vi "MDPtrMgr Info.vi"(8 "error in (no error)":errorcluster) -> (0 "error out":errorcluster, 1 "# free elements in queue":i32, 2 "# elements in queue":i32, 3 "Queue Names":string[](array[string]), 4 "#queues":i32)   [LabVIEW 2017, in "MDPtr.lvlib"]
uses:
  MDPtr.lvlib
  _MDPtrMgr/MDPtrMgr.lvclass
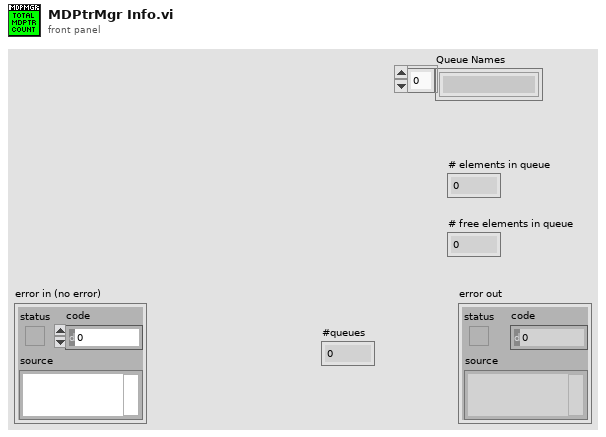
[diagram p1: front panel]
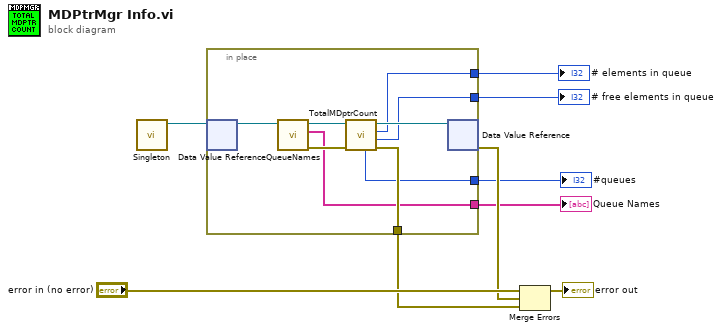
[diagram p0: block diagram]
diagram:
  n1 = call "Singleton.vi"() -> ("MDPtrMgrDVR"=w9:refnum<data-value>)  [unwired: 9 in, 2 out]
  n2 = in-place {
    in-place-border: [w17] -> w5
    in-place-border: [w16] -> w4
    in-place-border: [w15] -> w3
    in-place-border: [w14] -> w2
    in-place-border: [w10] -> w1
    n3 = in-place-dvr #1(w9) -> (w13:refnum<class "MDPtrMgr.lvclass">)  [unwired: 1 out]
    n4 = call "QueueNames.vi"("MDPtrMgr in"=w13) -> ("error out"=w11:errorcluster, "Queue Names"=w10:string[], "MDPtrMgr out"=w12:refnum<class "MDPtrMgr.lvclass">)  [unwired: 8 in]
    n5 = call "TotalMDptrCount.vi"("error in (no error)"=w11, "MDPtrMgr in"=w12) -> ("error out"=w17:errorcluster, "# free elements in queue"=w15:i32, "# elements in queue"=w16:i32, "MDPtrMgr out"=w18:refnum<class "MDPtrMgr.lvclass">, "#queues"=w14:i32)  [unwired: 5 in]
    n6 = in-place-dvr #1(w18) -> (w6:errorcluster)  [unwired: 1 out]
  }
  "# elements in queue" <- w4
  "# free elements in queue" <- w3
  "#queues" <- w2
  "Queue Names" <- w1
  n7 = Merge Errors("error in (no error)", w6, w5) -> (→"error out":errorcluster)
